vi "test bench_FXP_Linear_control_law.vi"() -> ()   [LabVIEW 2017]
uses:
  fpga_subVIs_ssxy/fixed-point-ss/typeDefs/FXPControlParams_distEst.ctl
  fpga_subVIs_ssxy/fixed-point-ss/typeDefs/x_vec_type.ctl
  fpga_subVIs_ssxy/fixed-point-ss/typeDefs/UT_matrix_data.ctl
  fpga_subVIs_ssxy/fixed-point-ss/typeDefs/Bz_vec_scalar.ctl
  fpga_subVIs_ssxy/fixed-point-ss/typeDefs/Lz_vec_scalar.ctl
  fpga_subVIs_ssxy/fixed-point-ss/typeDefs/Kz_vec_scalar.ctl
  fpga_subVIs_ssxy/fixed-point-ss/typeDefs/Nx_vec_scalar.ctl
  fpga_subVIs_ssxy/fixed-point-ss/typeDefs/Az_vec_scalar.ctl
  fpga_subVIs_ssxy/fixed-point-ss/typeDefs/x_vec_scalar.ctl
  fpga_subVIs_ssxy/fixed-point-ss/typeDefs/Cz_vec_scalar.ctl
  fpga_subVIs_ssxy/fixed-point-ss/typeDefs/x_vec_bram.ctl
  fpga_subVIs_ssxy/fixed-point-ss/typeDefs/Kz_bram.ctl
  <vilib>/rvi/Emulation/niFpgaEmulationIsFPGAContextNoSignature.vi
  <vilib>/rvi/DataTransferAndStorage/Container/Common/niFpgaContainerGetUniqueNameForEmu.vi
  <vilib>/rvi/Memory/Memory_Emulation/niFpgaMemoryEmulationCacheClearOnFirstRun.vi
  <vilib>/rvi/Memory/Memory_Emulation/nirvimemoryEmulationManagerCache_MakeExclusive.vi
  <vilib>/rvi/Memory/Memory_Emulation/niFpgaMemoryEmulationValidateCache.vi
  <vilib>/rvi/Memory/Memory_Emulation/nirvimemoryEmulationManagerCache_InsertValue.vi
  <vilib>/Utility/error.llb/Clear Errors.vi
  <vilib>/rvi/Memory/Memory_Emulation/nirvimemoryEmulationManagerCache_ReleaseExclusive.vi
  <vilib>/rvi/Memory/Memory_Emulation/nirvimemoryEmulationManagerCache_GetValue.vi
  <vilib>/rvi/Memory/Memory_Emulation/nirvimemoryEmulationManagerCache_SetValue.vi
  <vilib>/rvi/Emulation/niFpgaProcessEmulError.vi
  <vilib>/rvi/Emulation/niFpgaSctlEmulationGetInTimedLoop.vi
  <vilib>/rvi/DataTransferAndStorage/Container/Common/niFpgaContainerExecOnDevCompGetState.vi
  <vilib>/rvi/errors/nirviReportUnexpectedCaseInternalError (U32).vi
  <vilib>/rvi/Emulation/niFpgaSctlEmulationResourceMgr.vi
  <vilib>/rvi/DataTransferAndStorage/Container/XNode/niFpgaContainer.xnode
  <vilib>/rvi/DataTransferAndStorage/Register/Emulation/niFpgaRegisterEmulation.vi
  <vilib>/rvi/Memory/Memory_Emulation/niFpgaMemoryEmulationRefIn.vi
panel:
  in  "xu":fxp<+/-,32,6>
  in  "matrix data":T1
  out "xk_0_2 (out)":T9
  in  "xk_12":T9=[0.0, 0.0, 0.0, 0.0, 0.0, 0.0, 0.0, 0.0, 0.0, 0.0, 0.0, 0.0, 0.0, 0.0, 0.0, 0.0, 0.0, 0.0, 0.0, 0.0, 0.0, 0.0, 0.0, 0.0, 0.0]
  in  "yd_est":fxp<+/-,32,5>
  out "del u(k)":fxp<+/-,64,15>
  out "u_k (saturated)":fxp<+/-,32,5>
  in  "ControlParams_distEst":T10={"umax"=3.0, "Ns_obs/cntrl"=0, "ref_f_VEC"=[0.0, 0.0], "du_max"=0.0, "Nbar"=0.0}
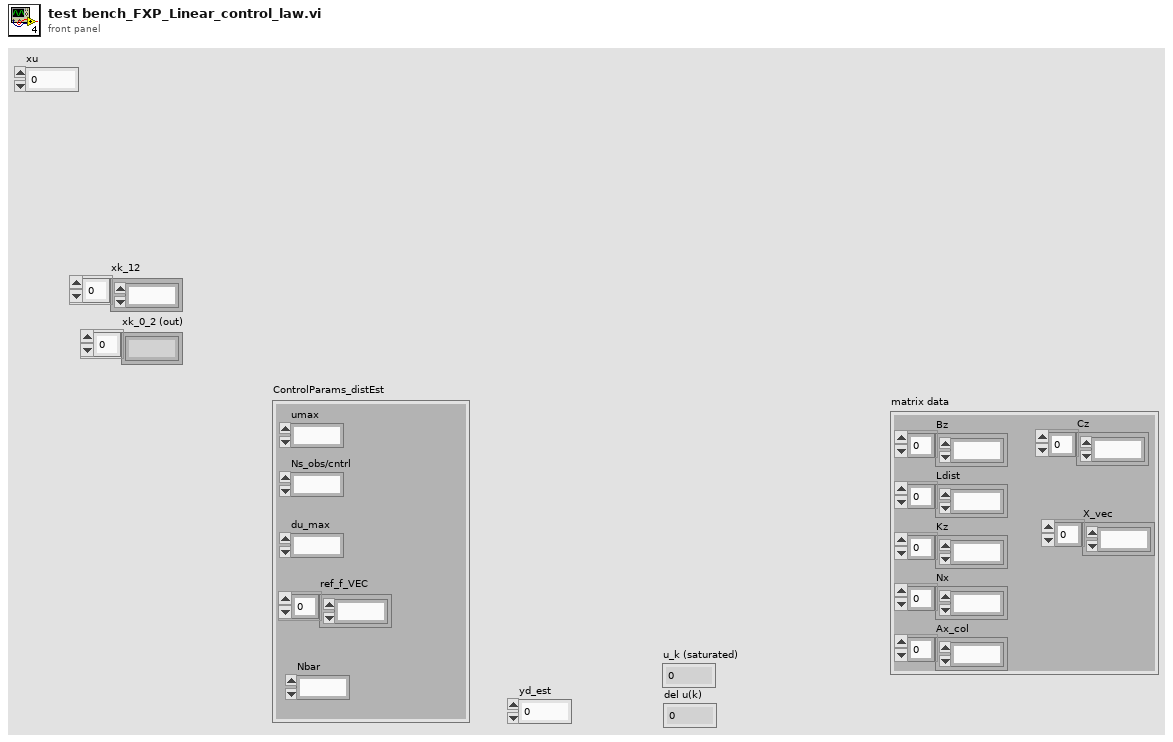
[diagram p1: front panel]
types:
  T1 = typedef "UT_matrix_data.ctl" = cluster{"Bz":T2[], "Ldist":T3[], "Kz":T4[], "Nx":T5[], "Ax_col":T6[], "X_vec":T7[], "Cz":T8[]}
  T2 = typedef "Bz_vec_scalar.ctl" = fxp<+/-,32,3>
  T3 = typedef "Lz_vec_scalar.ctl" = fxp<+/-,32,3>
  T4 = typedef "Kz_vec_scalar.ctl" = fxp<+/-,32,10>
  T5 = typedef "Nx_vec_scalar.ctl" = fxp<+/-,32,2>
  T6 = typedef "Az_vec_scalar.ctl" = fxp<+/-,32,7>
  T7 = typedef "x_vec_scalar.ctl" = fxp<+/-,32,6>
  T8 = typedef "Cz_vec_scalar.ctl" = fxp<+/-,32,4>
  T9 = typedef "x_vec_type.ctl" = fxp<+/-,32,6>[]
  T10 = typedef "FXPControlParams_distEst.ctl" = cluster{"umax":fxp<+/-,18,5>, "Ns_obs/cntrl":u8, "ref_f_VEC":fxp<+/-,32,5>[], "du_max":fxp<+/-,18,5>, "Nbar":fxp<+/-,32,5>}
  T11 = typedef "x_vec_bram.ctl" = refnum<k21>
  T12 = typedef "Kz_bram.ctl" = refnum<k21>
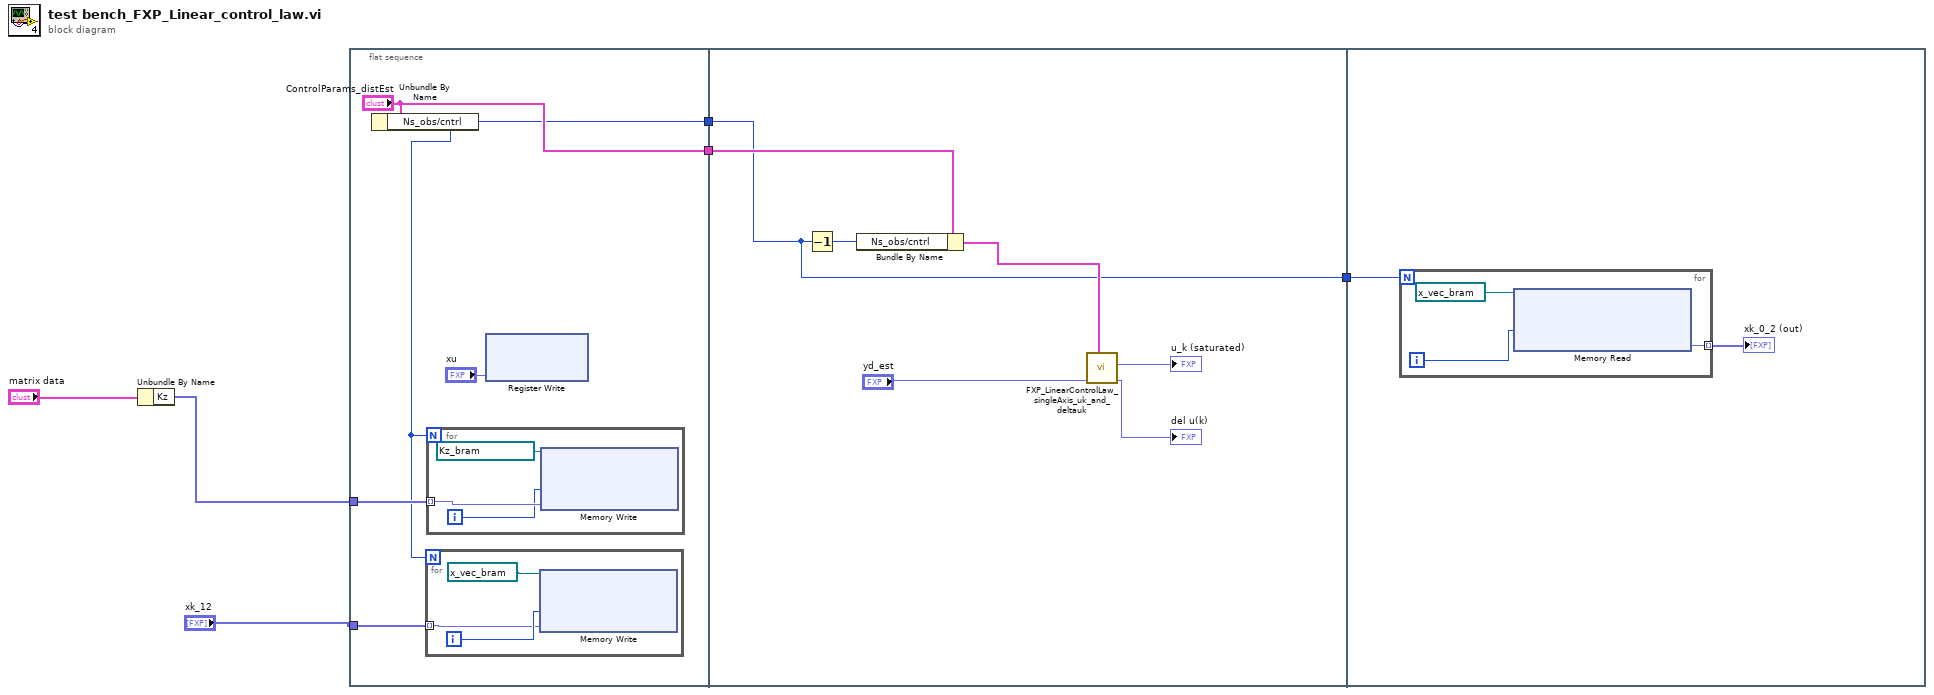
[diagram p0: block diagram]
diagram:
  n1 = Unbundle By Name("matrix data") -> ("Kz"=w3:T4[])
  n2 = flat-sequence {
    tunnel: ["ControlParams_distEst"] -> w5
    tunnel: [w8] -> w4
    tunnel: w3 -> [w10]
    tunnel: "xk_12" -> [w9]
    tunnel: [w18] -> w6
    tunnel: w5 -> [w24]
    tunnel: w4 -> [w18]
    tunnel: w6 -> [w26]
    frame #0 {
      n3 = Unbundle By Name("ControlParams_distEst") -> ("Ns_obs/cntrl"=w8:u8)
      n4 = for {
        N: w8 -> [_]
        tunnel: w9 -> [w13] mode=indexing
        i -> [w14]
        n5 = xnode "Memory Write"("Address"=w14, "Data"=w13, "Memory In"=T11 "xk_0_2" ("Memory")) -> ()  [unwired: 1 out]
      }
      n6 = for {
        N: w8 -> [_]
        tunnel: w10 -> [w17] mode=indexing
        i -> [w16]
        n7 = xnode "Memory Write"("Address"=w16, "Data"=w17, "Memory In"=T12 "K_FXP_row1" ("Memory")) -> ()  [unwired: 1 out]
      }
      n8 = xnode "Register Write"("Data"="xu") -> ()  [unwired: 1 in, 1 out]
    }
    frame #1 {
      n9 = Decrement(x=w18) -> (x-1=w23:u8)
      n10 = Bundle By Name(cluster=w24, "Ns_obs/cntrl"=w23) -> (w19:T10)
      n11 = call "FXP_LinearControlLaw_singleAxis_uk_and_deltauk.vi"("ControlParams_distEst"=w19, "yd_est_x"="yd_est") -> ("del u_x"=→"del u(k)":fxp<+/-,64,15>, "u_k (un saturated)"=→"u_k (saturated)":fxp<+/-,32,5>)  [unwired: 8 in]
    }
    frame #2 {
      n12 = for {
        N: w26 -> [_]
        tunnel: [w28] -> w25 mode=indexing
        i -> [w29]
        n13 = xnode "Memory Read"("Address"=w29, "Memory In"=T11 "xk_0_2" ("Memory")) -> ("Data"=w28:fxp<+/-,32,6>)  [unwired: 1 out]
      }
      "xk_0_2 (out)" <- w25
    }
  }
